vi "checkFinishBallPlacementAllyPlay.vi"(8 "error in (no error)":errorcluster, 10 "Game":refnum<class "Game.lvclass">, 11 "BallPlacementAllyPlay in":refnum<class "BallPlacementAllyPlay.lvclass">) -> (0 "error out":errorcluster, 2 "finishBallPlacementAlly":bool, 3 "BallPlacementAllyPlay out":refnum<class "BallPlacementAllyPlay.lvclass">)   [LabVIEW 2021, in "BallPlacementAllyPlay.lvclass"]
uses:
  BallPlacementAllyPlay.lvclass
  Game_class/Game.lvclass
  Game_class/Game.lvclass/Game.ctl
  Referee_class/command_interpreted.ctl
  Robot_class/roles.ctl
  Referee_class/Referee.lvclass/Referee.ctl
  Ball_class/Ball.lvclass/Ball.ctl
  Object_class/Object.lvclass/Object.ctl
  Team_class/Team.lvclass/Team.ctl
  <vilib>/Analysis/_algsub.llb/Real Vector Norm.vi
  Game_class/Read BallRef.vi
  Game_class/Read KeeperTeam.vi
  Game_class/Read Utilities.lvclass.vi
  Team_class/Read RobotRef.vi
  Ball_class/Read v_x.vi
  Ball_class/Read v_y.vi
  Object_class/Read position(x,y).vi
  Referee_class/Read command_interpreted.vi
  Game_class/Read Referee.vi
  Ally_class/Ally.lvclass
  D:/RoboIme/horie/SSL_AI/Team_class/Team.lvclass
  Ball_class/Ball.lvclass
  D:/RoboIme/horie/SSL_AI/Object_class/Object.lvclass
  Referee_class/Referee.lvclass
  Utilities_class/Utilities.lvclass
  Robot_class/Robot.lvclass
  <vilib>/Analysis/NI_AALPro.lvlib
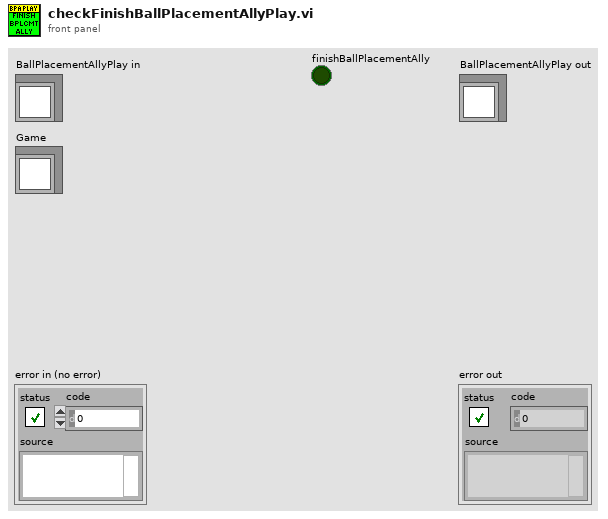
[diagram p1: front panel]
types:
  T1 = typedef "roles.ctl" = enum16{"SimpleBallPlacement", "BallPlacementAllyPasser", "BallPlacementAllyReceiver", "BallPlacementEnemy", "5Robots5th", "PassBestReceiver", "5Robots4th", "5Robots3rd", "5Robots2nd", "5Robots1st", "PassBestRobot", "WaitPass", "ABCThirdKicker", "ABCFirstKicker", "ABCSecondKicker", "Tabler", "TableFinalizer", "PrepareRollToPassRoller", "PrepareRollToPassReceiver", "SimplePassRoll", "SimplePassRollReceiver", "PenaltyDefense", "PreparePassReceiver 2", "PreparePassReceiver 1", "PassObserver", "Timeout", "Goto", "ZigZag", "None", "BallOutOfField", "DefenderArea", "Duelist", "AttackerStop", "FollowAttacker", "KeeperRole", "KickPenalty", "AttackerAimGoal", "AttackerBlock", "Marker", "Halt", "Shoot", "PassKicker", "PassReceiver", "TestRole", "PenaltyAttacker"}
  T2 = typedef "command_interpreted.ctl" = enum16{"Goal Ally", "Goal Enemy", "Ball Placement Enemy", "Ball Placement Ally", "Normal Half Time", "Extra Time  Break", "Extra Half Time", "None", "Post Game", "PKA Normal Start", "Prepare Kickoff Ally", "PKE Normal Start", "Prepare Kickoff Enemy", "Force Start", "Halt", "Timeout", "Prepare Penalty Ally", "Prepare Penalty Enemy", "PPA NormalStart", "PPE Normal Start", "Indirect Free Ally", "Direct Free Enemy", "Direct Free Ally", "Indirect Free Enemy", "Stop"}
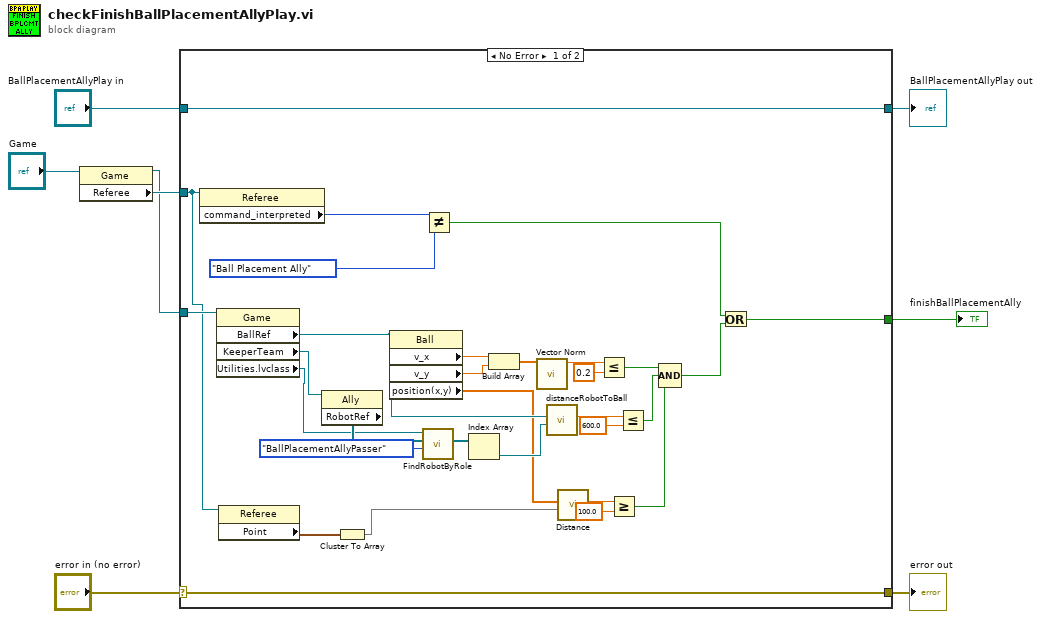
[diagram p0: block diagram]
diagram:
  n1 = property class="Game"(reference="Game") -> (reference out=w1:refnum<class "Game.lvclass">, "Referee"=w2:refnum<class "Referee.lvclass">)  [unwired: 1 in, 1 out]
  n2 = case shown="No Error" "error in (no error)" {
    selector: "error in (no error)" -> [w38 w41]
    tunnel: [w38 w41] -> w7
    tunnel: [w39 w40] -> w5
    tunnel: "BallPlacementAllyPlay in" -> [w39 w40]
    tunnel: w2 -> [w14 _]
    tunnel: [w18 _] -> w4
    tunnel: w1 -> [w15 _]
    frame No Error {
      n3 = property class="Referee"(reference=w14) -> ("command_interpreted"=w37:T2)  [unwired: 1 in, 2 out]
      n4 = property class="Game"(reference=w15) -> ("BallRef"=w28:refnum<class "Ball.lvclass">, "KeeperTeam"=w23:refnum<class "Ally.lvclass">, "Utilities.lvclass"=w17:refnum<class "Utilities.lvclass">)  [unwired: 1 in, 2 out]
      n5 = property class="Referee"(reference=w14) -> ("Point"=w13:cluster{"x":sgl, "y":sgl})  [unwired: 1 in, 2 out]
      n6 = property class="Ally"(reference=w23) -> ("RobotRef"=w22:refnum<class "Robot.lvclass">[])  [unwired: 1 in, 2 out]
      n7 = Cluster To Array(cluster=w13) -> (array=w12:sgl[])
      n8 = property class="Ball"(reference=w28) -> ("v_x"=w34:dbl, "v_y"=w33:dbl, "position(x,y)"=w16:dbl[])  [unwired: 1 in, 2 out]
      n9 = call "FindRobotByRole.vi"("role"=roles."BallPlacementAllyPasser", "RobotRef"=w22, "Utilities in"=w17) -> ("Robots"=w27:refnum<class "Robot.lvclass">[])  [unwired: 6 in, 2 out]
      n10 = Not Equal?(x=w37, y=command_interpreted."Ball Placement Ally") -> (x != y?=w35:bool)
      n11 = Index Array(array=w27) -> (element=w26:refnum<class "Robot.lvclass">)  [unwired: 1 in]
      n12 = Build Array(w34, w33) -> (w32:dbl[])
      n13 = call-poly <vilib>:"Vector Norm.vi"("Input Vector"=w32) -> ("norm"=w31:dbl)  [unwired: 9 in, 1 out]
      n14 = call "distanceRobotToBall.vi"("Robot"=w26, "Ball"=w28) -> ("Distance Robot To Ball"=w25:dbl)  [unwired: 7 in, 2 out]
      n15 = call "Distance.vi"("P1"=w12, "P2"=w16) -> ("Distance"=w11:dbl)  [unwired: 7 in, 2 out]
      n16 = Less Or Equal?(x=w31, y=0.2) -> (x <= y?=w29:bool)
      n17 = Greater Or Equal?(x=w11, y=100.0) -> (x >= y?=w9:bool)
      n18 = Less Or Equal?(x=w25, y=600.0) -> (x <= y?=w20:bool)
      n19 = Compound Arithmetic op=AND(w29, w20, w9) -> (w19:bool)
      n20 = Or(x=w35, y=w19) -> (x .or. y?=w18:bool)
    }
    frame Error {
    }
  }
  "error out" <- w7
  "BallPlacementAllyPlay out" <- w5
  "finishBallPlacementAlly" <- w4
